vi "Convert C to F.vi"() -> ()   [LabVIEW 2015]
doc: "This is a cool vi program to convert temperature from degree centigrade to fahrenheit."
panel:
  out "deg F":dbl(slide) scale=0.0..300.0
  in  "deg C":dbl(slide) scale=0.0..100.0
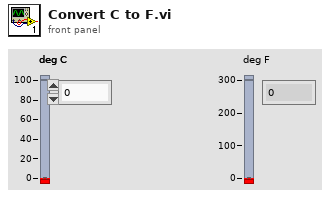
[diagram p1: front panel]
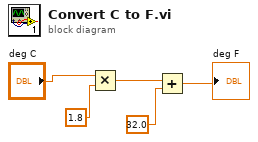
[diagram p0: block diagram]
diagram:
  n1 = Multiply(x="deg C", y=1.8) -> (x*y=w3:dbl)
  n2 = Add(x=w3, y=32.0) -> (x+y=→"deg F":dbl)
